vi "populate_map.vi"(8 "error in (no error)":errorcluster, 10 "variable_info_in":T3, 11 "IO_variable_map_in":T1[](array[typedef])) -> (0 "error out":errorcluster, 3 "IO_variable_map_out":T1[](array[typedef]))   [LabVIEW 2015, in "Scan Engine runtime.lvclass"]
uses:
  Scan Engine runtime.lvclass
  Custom Ctrls/Index Map.ctl
  <vilib>/NI/Tag Bus/tag/Data Type.ctl
  Custom Ctrls/IO_index_map.ctl
  <vilib>/NI/Tag Bus/tag/tag descriptor.lvclass
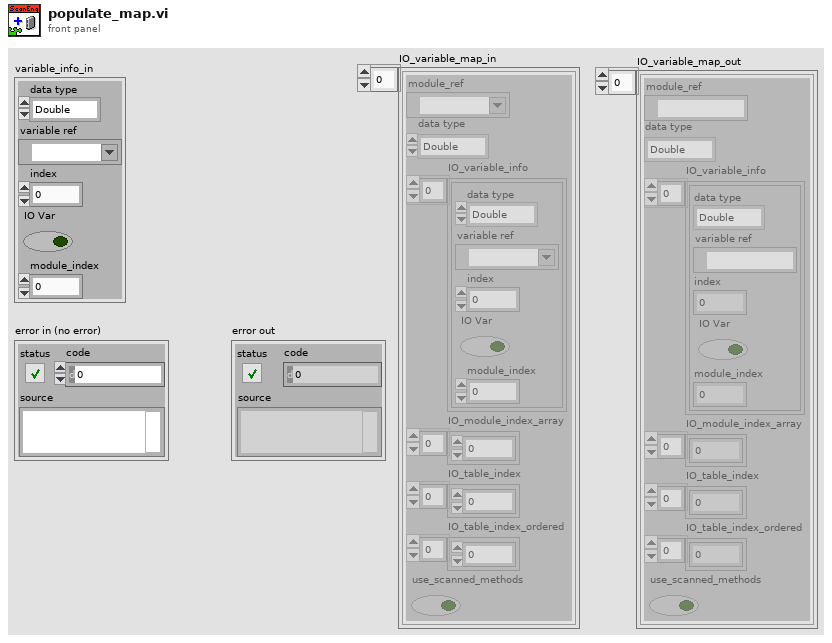
[diagram p1: front panel]
types:
  T1 = typedef "Scan Engine runtime.lvclass/IO_index_map.ctl" = cluster{"module_ref":refnum<k21>, "data type":T2, "IO_variable_info":T3[], "IO_module_index_array":i32[], "IO_table_index":i32[], "IO_table_index_ordered":i32[], "use_scanned_methods":bool}
  T2 = typedef "tag bus.lvlib/tag descriptor.lvclass/Data Type.ctl" = enum16{"Double", "Single", "I64", "I32", "I16", "I8", "U64", "U32", "U16", "U8", "Boolean", "String", "Array of Double", "Array of Single", "Array of I64", "Array of I32", "Array of I16", "Array of I8", "Array of U64", "Array of U32", "Array of U16", "Array of U8", "Array of Boolean", "Array of String"}
  T3 = typedef "Scan Engine runtime.lvclass/Index Map.ctl" = cluster{"data type":T2, "variable ref":refnum<k21>, "index":i32, "IO Var":bool, "module_index":i32}
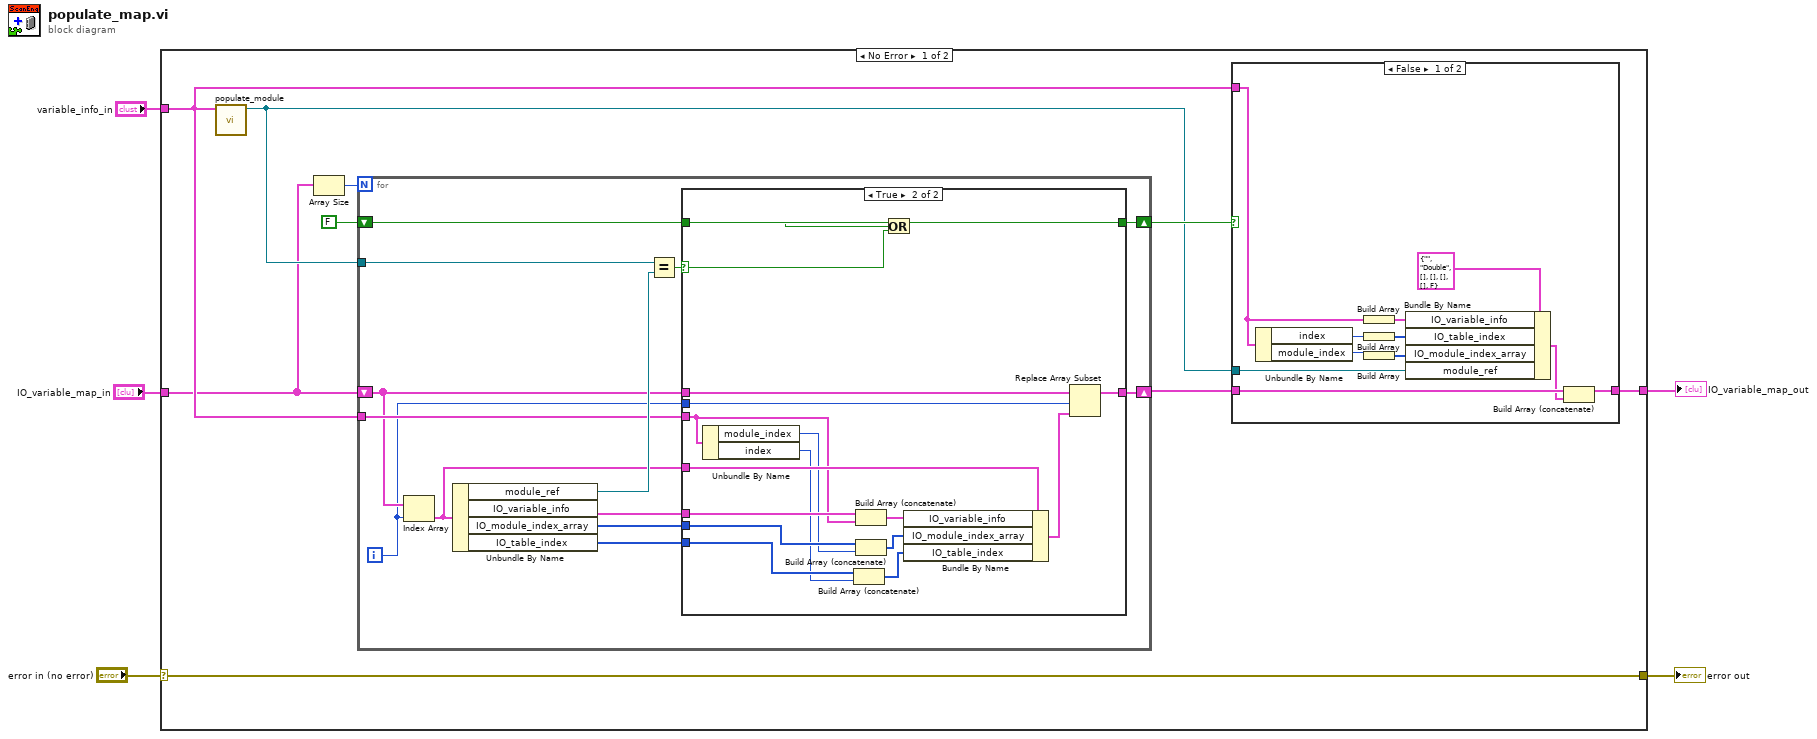
[diagram p0: block diagram]
diagram:
  n1 = case shown="No Error" "error in (no error)" {
    selector: "error in (no error)" -> [w6 w60]
    tunnel: "variable_info_in" -> [w10 _]
    tunnel: "IO_variable_map_in" -> [w8 w59]
    tunnel: [w7 w59] -> w3
    tunnel: [w6 w60] -> w1
    frame No Error {
      n2 = call "populate_module.vi"("variable_info_in"=w10) -> ("Module"=w9:refnum<k21>)  [unwired: 10 in]
      n3 = Array Size(array=w8) -> (size(s)=w14:i32)
      n4 = for {
        N: w14 -> [_]
        tunnel: w9 -> [w39]
        tunnel: w10 -> [w36]
        shift-right: [w32] -> w11
        shift-left: w8 -> [w35]
        shift-right: [w29] -> w12
        shift-left: FALSE -> [w30]
        i -> [w33]
        n5 = Index Array(array=w35, index=w33) -> (element=w34:T1)
        n6 = Unbundle By Name(w34) -> ("module_ref"=w38:refnum<k21>, "IO_variable_info"=w37:T3[], "IO_module_index_array"=w28:i32[], "IO_table_index"=w27:i32[])
        n7 = Equal?(x=w39, y=w38) -> (x = y?=w31:bool)
        n8 = case shown="True" w31 {
          selector: w31 -> [_ w51]
          tunnel: w37 -> [_ w58]
          tunnel: w36 -> [_ w47]
          tunnel: w35 -> [w41 w57]
          tunnel: w34 -> [_ w56]
          tunnel: w33 -> [_ w55]
          tunnel: [w41 w54] -> w32
          tunnel: w30 -> [w40 w52]
          tunnel: [w40 w50] -> w29
          tunnel: w28 -> [_ w48]
          tunnel: w27 -> [_ w43]
          frame False {
          }
          frame True {
            n9 = Unbundle By Name(w47) -> ("module_index"=w46:i32, "index"=w42:i32)
            n10 = Build Array (concatenate)(w43, w42) -> (w44:i32[])
            n11 = Build Array (concatenate)(w58, w47) -> (w49:T3[])
            n12 = Build Array (concatenate)(w48, w46) -> (w45:i32[])
            n13 = Or(x=w52, y=w51) -> (x .or. y?=w50:bool)
            n14 = Bundle By Name(cluster=w56, "IO_variable_info"=w49, "IO_module_index_array"=w45, "IO_table_index"=w44) -> (w53:T1)
            n15 = Replace Array Subset(array=w57, new element=w53, index=w55) -> (w54:T1[])
          }
        }
      }
      n16 = case shown="False" w12 {
        tunnel: w11 -> [w25 w26]
        tunnel: [w24 w26] -> w7
        tunnel: w9 -> [w16 _]
        tunnel: w10 -> [w21 _]
        frame False {
          n17 = Unbundle By Name(w21) -> ("index"=w18:i32, "module_index"=w19:i32)
          n18 = Build Array(w21) -> (w17:T3[])
          n19 = Build Array(w18) -> (w15:i32[])
          n20 = Build Array(w19) -> (w20:i32[])
          n21 = Bundle By Name(cluster=T1 {"module_ref"="", "data type"=enum."Double", "IO_variable_info"=[], "IO_module_index_array"=[], "IO_table_index"=[], "IO_table_index_ordered"=[], "use_scanned_methods"=FALSE} ("IO_variables_per_module"), "IO_variable_info"=w17, "IO_table_index"=w15, "IO_module_index_array"=w20, "module_ref"=w16) -> (w23:T1)
          n22 = Build Array (concatenate)(w25, w23) -> (w24:T1[])
        }
        frame True {
        }
      }
    }
    frame Error {
    }
  }
  "IO_variable_map_out" <- w3
  "error out" <- w1
